vi "Discharge_C108_C109.vi"(8 "error in (no error)":errorcluster, 10 "Parameters":string, 11 "reference in":refnum<class "Test_Flux_Capacitor.lvclass">) -> (0 "error out":errorcluster, 2 "Result":bool, 3 "reference out":refnum<class "Test_Flux_Capacitor.lvclass">)   [LabVIEW 2022 SP3, in "Test_Flux_Capacitor.lvlib" / "Test_Flux_Capacitor.lvclass"]
uses:
  Test_Flux_Capacitor.lvclass
  ParameterTypes/Discharge_C108_C109.ctl
  <vilib>/Utility/error.llb/Trim Whitespace One-Sided.vi
  Components/SwitchBase.lvlibp/SwitchBase.lvclass
  <vilib>/JDP Science/JSONtext/JSONtext.lvlib
panel:
  in  "Parameter_Type":T1
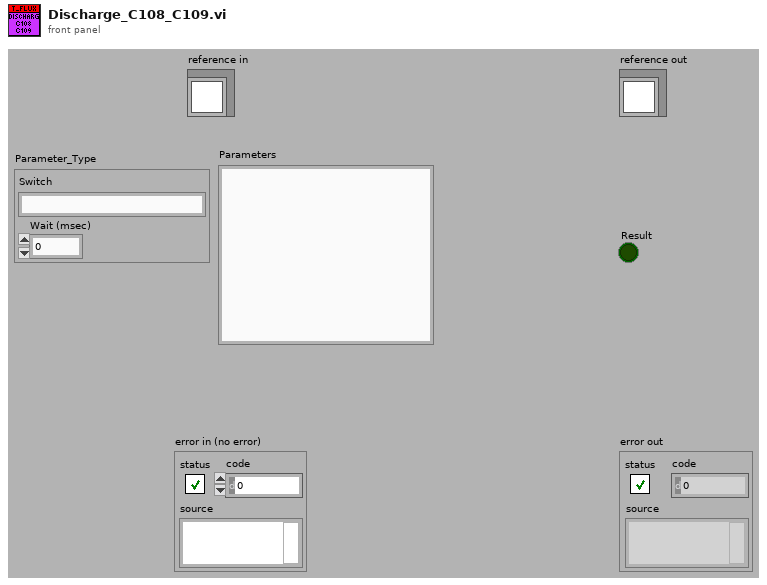
[diagram p1: front panel]
types:
  T1 = typedef "Test_Flux_Capacitor.lvlib/Test_Flux_Capacitor.lvclass/Discharge_C108_C109.ctl" = cluster{"Switch":string, "Wait (msec)":u32}
  T2 = typedef "Test_Flux_Capacitor.lvlib/Test_Flux_Capacitor.lvclass/ObjectAttributes.ctl" = cluster{"Config":T3, "DMM":refnum<class "DMM_Keysight_34980A.lvclass">, "LCR":refnum<class "LCR_BK891.lvclass">, "PSU":refnum<class "PSU_Base.lvclass">, "Switch_Manager":refnum<class "SwitchBase.lvclass">, "FRAM":string, "Flux_Capacitor":refnum<class "Flux_Capacitor.lvclass">, "Frequency_Counter":refnum<class "Frequency_Counter_Base.lvclass">, "JTAG":refnum<class "JTAG_Base.lvclass">}
  T3 = typedef "Test_Flux_Capacitor.lvlib/Test_Flux_Capacitor.lvclass/Config.ctl" = cluster{"default":string}
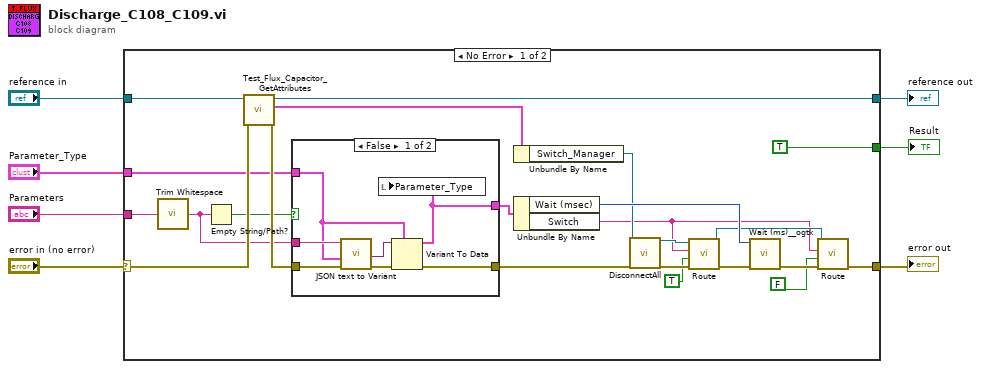
[diagram p0: block diagram]
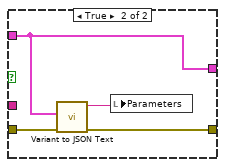
[diagram p2: hidden frame]
diagram:
  n1 = case shown="No Error" "error in (no error)" {
    selector: "error in (no error)" -> [w30 w43]
    tunnel: [w20 w43] -> w6
    tunnel: [w28 w42] -> w4
    tunnel: "reference in" -> [w29 w42]
    tunnel: "Parameters" -> [w17 _]
    tunnel: "Parameter_Type" -> [w25 _]
    tunnel: [TRUE _] -> w2
    frame No Error {
      n2 = call <vilib>:"Trim Whitespace.vi"("string"=w17) -> ("trimmed string"=w16:string)  [unwired: 1 in]
      n3 = Empty String/Path?(string/path=w16) -> (empty?=w15:bool)
      n4 = call "Test_Flux_Capacitor_GetAttributes.vi"("error in (no error)"=w30, "reference in"=w29) -> ("error out"=w26:errorcluster, "Data"=w27:T2, "reference out"=w28:refnum<class "Test_Flux_Capacitor.lvclass">)  [unwired: 6 in, 1 out]
      n5 = case shown="False" w15 {
        tunnel: w26 -> [w35 w41]
        tunnel: w25 -> [w32 w40]
        tunnel: [w37 w38] -> w14
        tunnel: [w36 w40] -> w18
        tunnel: w16 -> [w33 _]
        frame False {
          n6 = call <vilib>:"JSON text to Variant.vi"("error in (no error)"=w35, "Data Type"=w32, "JSON"=w33) -> ("error out"=w34:errorcluster, "Variant out"=w31:variant)  [unwired: 7 in]
          n7 = Variant To Data(error in=w34, type=w32, Variant=w31) -> (data=w36:T1, error out=w37:errorcluster)
          n8 = local write "Parameter_Type"(w36) -> ()
        }
        frame True {
          n9 = call <vilib>:"Variant to JSON Text.vi"("error in (no error)"=w41, "Variant"=w40) -> ("error out"=w38:errorcluster, "<JSON>"=w39:string)  [unwired: 7 in, 1 out]
          n10 = local write "Parameters"(w39) -> ()
        }
      }
      n11 = Unbundle By Name(w27) -> ("Switch_Manager"=w12:refnum<class "SwitchBase.lvclass">)
      n12 = Unbundle By Name(w18) -> ("Wait (msec)"=w23:u32, "Switch"=w9:string)
      n13 = call-dynamic "DisconnectAll.vi"("reference in"=w12, "error in (no error)"=w14) -> ("reference in"=w11:refnum<class "SwitchBase.lvclass">, "error out"=w13:errorcluster)  [unwired: 16 in]
      n14 = call-dynamic "Route.vi"("error in (no error)"=w13, "Connect"=TRUE, "channel 1"=w9, "reference in"=w11) -> ("error out"=w24:errorcluster, "reference in"=w22:refnum<class "SwitchBase.lvclass">)  [unwired: 6 in]
      n15 = call <userlib>:"Wait (ms)__ogtk.vi"("error in (no error)"=w24, "milliseconds to wait"=w23) -> ("error out"=w21:errorcluster)  [unwired: 8 in, 1 out]
      n16 = call-dynamic "Route.vi"("error in (no error)"=w21, "Connect"=FALSE, "channel 1"=w9, "reference in"=w22) -> ("error out"=w20:errorcluster)  [unwired: 6 in, 1 out]
    }
    frame Error {
    }
  }
  "Result" <- w2
  "error out" <- w6
  "reference out" <- w4
